vi "Init Tooltip and Description.vi"(10 "Supported Devices":u32[](array[numeric]), 11 "Main UI Ref Cluster":T1) -> ()   [LabVIEW 2021, in "myRIOMetaDataObj.lvclass"]
uses:
  myRIOMetaDataObj.lvclass
  WizardUIRef.ctl
  AvailableTargets.ctl
  Tooltip and Description Message.vi
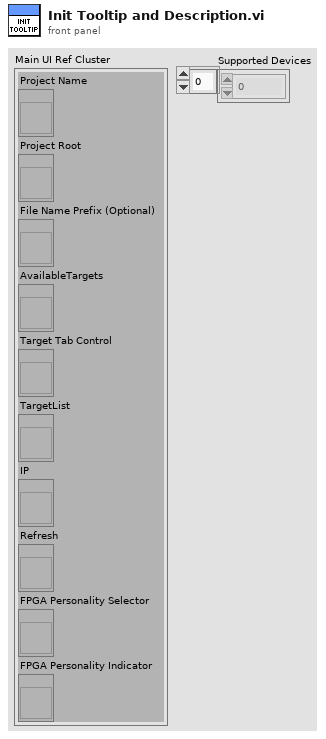
[diagram p1: front panel]
types:
  T1 = typedef "myRIOMetaDataObj.lvclass/WizardUIRef.ctl" = cluster{"Project Name":refnum<vi>, "Project Root":refnum<vi>, "File Name Prefix (Optional)":refnum<vi>, "AvailableTargets":refnum<vi>, "Target Tab Control":refnum<vi>, "TargetList":refnum<vi>, "IP":refnum<vi>, "Refresh":refnum<vi>, "FPGA Personality Selector":refnum<vi>, "FPGA Personality Indicator":refnum<vi>}
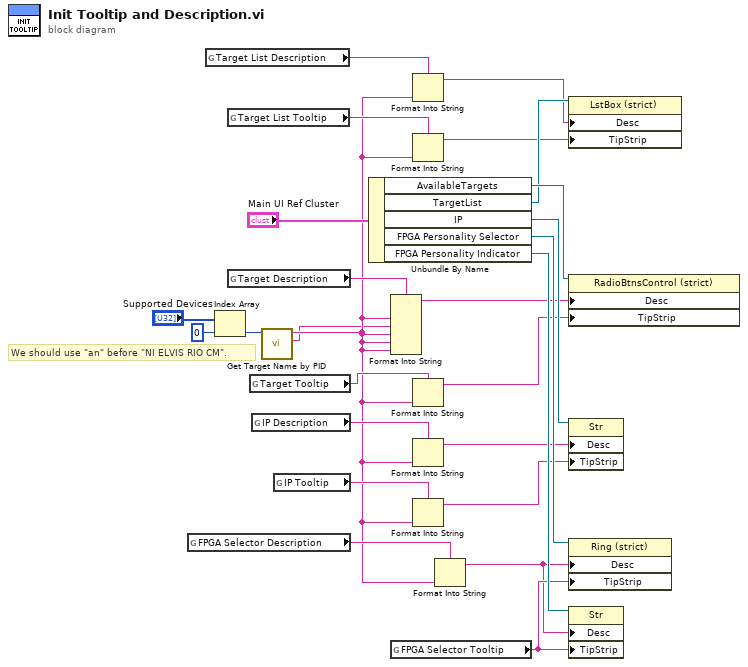
[diagram p0: block diagram]
diagram:
  # "We should use \"an\" before \"NI ELVIS RIO CM\"."
  n1 = global read "Tooltip and Description Message.vi" "FPGA Selector Description"() -> (w10:string)
  n2 = global read "Tooltip and Description Message.vi" "Target List Description"() -> (w16:string)
  n3 = Index Array(array="Supported Devices", index=0) -> (element=w4:u32)
  n4 = global read "Tooltip and Description Message.vi" "Target List Tooltip"() -> (w14:string)
  n5 = global read "Tooltip and Description Message.vi" "Target Description"() -> (w3:string)
  n6 = global read "Tooltip and Description Message.vi" "Target Tooltip"() -> (w17:string)
  n7 = global read "Tooltip and Description Message.vi" "IP Description"() -> (w12:string)
  n8 = call <vilib>:"Get Target Name by PID.vi"("Device Model"=w4) -> ("Article"=w1:string, "Device Model Str"=w2:string)  [unwired: 9 in]
  n9 = global read "Tooltip and Description Message.vi" "IP Tooltip"() -> (w11:string)
  n10 = Unbundle By Name("Main UI Ref Cluster") -> ("AvailableTargets"=w25:refnum<vi>, "TargetList"=w24:refnum<vi>, "IP"=w23:refnum<vi>, "FPGA Personality Selector"=w22:refnum<vi>, "FPGA Personality Indicator"=w21:refnum<vi>)
  n11 = Format Into String(format string=w3, w2, w1, w2, w2, w2) -> (resulting string=w18:string)  [unwired: 2 in, 1 out]
  n12 = global read "Tooltip and Description Message.vi" "FPGA Selector Tooltip"() -> (w9:string)
  n13 = Format Into String(format string=w16, w2) -> (resulting string=w15:string)  [unwired: 2 in, 1 out]
  n14 = Format Into String(format string=w14, w2) -> (resulting string=w13:string)  [unwired: 2 in, 1 out]
  n15 = Format Into String(format string=w17, w2) -> (resulting string=w7:string)  [unwired: 2 in, 1 out]
  n16 = Format Into String(format string=w12, w2) -> (resulting string=w6:string)  [unwired: 2 in, 1 out]
  n17 = Format Into String(format string=w11, w2) -> (resulting string=w5:string)  [unwired: 2 in, 1 out]
  n18 = Format Into String(format string=w10, w2) -> (resulting string=w8:string)  [unwired: 2 in, 1 out]
  n19 = property class="LstBox (strict)"(reference=w24, "Desc"=w15, "TipStrip"=w13) -> ()  [unwired: 1 in, 2 out]
  n20 = property class="RadioBtnsControl (strict)"(reference=w25, "Desc"=w18, "TipStrip"=w7) -> ()  [unwired: 1 in, 2 out]
  n21 = property class="Str"(reference=w23, "Desc"=w6, "TipStrip"=w5) -> ()  [unwired: 1 in, 2 out]
  n22 = property class="Ring (strict)"(reference=w22, "Desc"=w8, "TipStrip"=w9) -> ()  [unwired: 1 in, 2 out]
  n23 = property class="Str"(reference=w21, "Desc"=w8, "TipStrip"=w9) -> ()  [unwired: 1 in, 2 out]
